vi "fgv_erp42_data.vi"(7 "cmd":enum16{"init", "read", "write"}(ring), 11 "erp recv str":string) -> (1 "erp recv out":string, 2 "ERP_Receive out":T1, 3 "val":bool)   [LabVIEW 2019]
uses:
  Ctrl/erp42_receive_packet.ctl
panel:
  out "ERP_Receive":T1
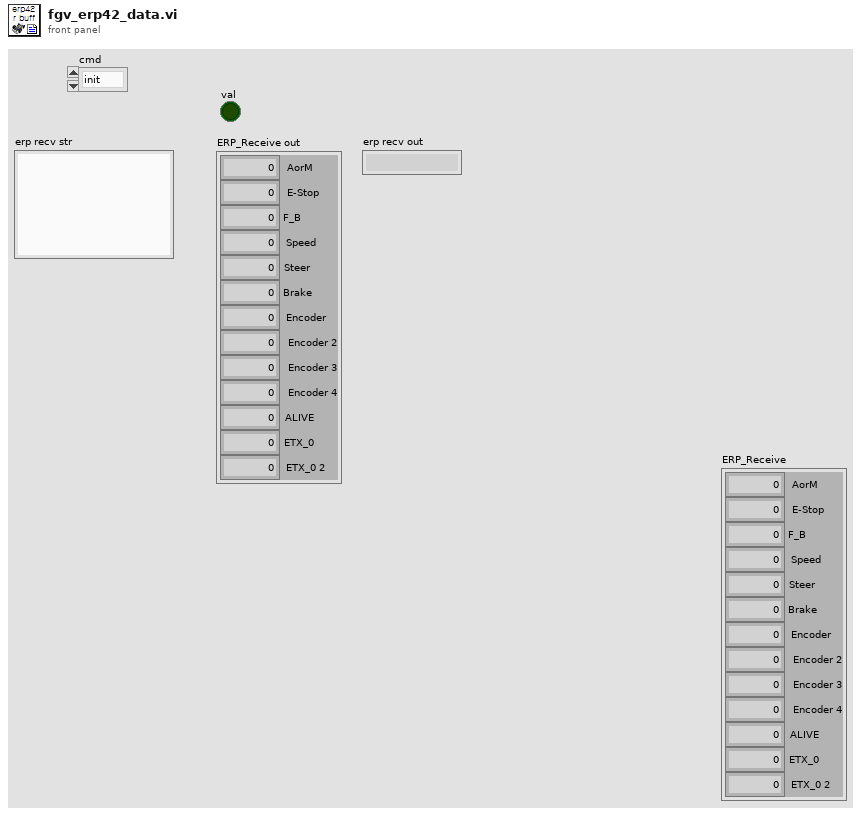
[diagram p1: front panel]
types:
  T1 = typedef "erp42_receive_packet.ctl" = cluster{"AorM":u8, "E-Stop":u8, "F_B":u8, "Speed":u16, "Steer":i16, "Brake":u8, "Encoder":u8, "Encoder 2":u8, "Encoder 3":u8, "Encoder 4":u8, "ALIVE":u8, "ETX_0":u8, "ETX_0 2":u8}
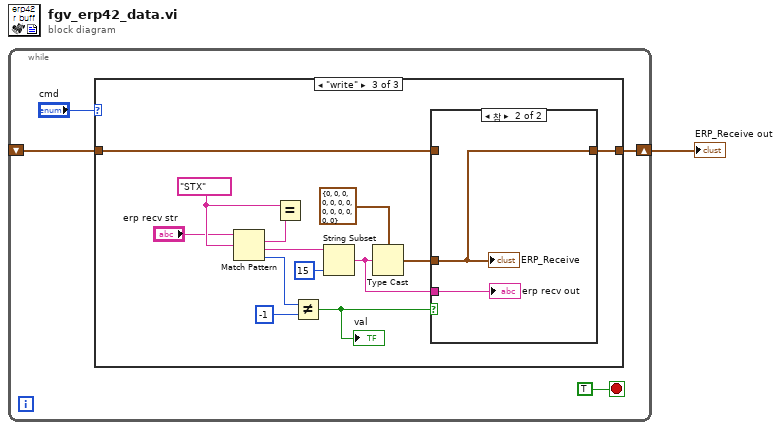
[diagram p0: block diagram]
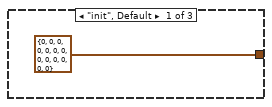
[diagram p2: hidden frame]
diagram:
  n1 = while {
    shift-right: [w3] -> w1
    shift-left: _ -> [w2]
    stop <- TRUE stop-if-true
    n2 = case shown="\"write\"" "cmd" {
      tunnel: [T1 {"AorM"=0, "E-Stop"=0, "F_B"=0, "Speed"=0, "Steer"=0, "Brake"=0, "Encoder"=0, "Encoder 2"=0, "Encoder 3"=0, "Encoder 4"=0, "ALIVE"=0, "ETX_0"=0, "ETX_0 2"=0} ("ERP_Receive") w7 w10] -> w3
      tunnel: w2 -> [_ w7 w9]
      frame "init", Default {
      }
      frame "read" {
      }
      frame "write" {
        w18 = "STX" ("검색 문자열/문자 (-)")
        n3 = Match Pattern(string="erp recv str", regular expression=w18) -> (match substring=w20:string, after substring=w19:string, offset past match=w14:i32)  [unwired: 1 in, 1 out]
        n4 = Equal?(x=w18, y=w20) -> ()  [unwired: 1 out]
        n5 = Not Equal?(x=w14, y=-1) -> (x != y?=w11:bool)
        "val" <- w11
        n6 = String Subset(string=w19, length (rest)=15 ("길이(나머지)")) -> (substring=w8:string)  [unwired: 1 in]
        n7 = Type Cast(type=T1 {"AorM"=0, "E-Stop"=0, "F_B"=0, "Speed"=0, "Steer"=0, "Brake"=0, "Encoder"=0, "Encoder 2"=0, "Encoder 3"=0, "Encoder 4"=0, "ALIVE"=0, "ETX_0"=0, "ETX_0 2"=0} ("ERP_Receive 3"), x=w8) -> (*(type *) &x=w12:T1)
        n8 = case shown="참" w11 {
          tunnel: w12 -> [_ w23]
          tunnel: [w21 w23] -> w10
          tunnel: w9 -> [w21 _]
          tunnel: w8 -> [_ w22]
          frame False {
          }
          frame True {
            "ERP_Receive" <- w23
            "erp recv out" <- w22
          }
        }
      }
    }
  }
  "ERP_Receive out" <- w1
